vi "movimentacao_cin_inv_cubo_magico.vi"() -> ()   [LabVIEW 2017]
doc: "The myRIO Project template acquires acceleration data from the onboard accelerometer and displays the changes of acceleration values in a waveform chart."
uses:
  <vilib>/Analysis/Matrix/Datatypes/RealMatrix.ctl
  <vilib>/myRIO/Instrument Drivers/Onboard IO/PWM/typedefs/PWM Reference.ctl
  <vilib>/myRIO/Common/Instrument Driver Framework/Utilities/typedefs/myRIO Generic Hardware Reference.ctl
  <vilib>/myRIO/Common/Instrument Driver Framework/Utilities/typedefs/Hardware Version Enum.ctl
  <vilib>/myRIO/Common/Instrument Driver Framework/Utilities/typedefs/myRIO v1.0 Reference.ctl
  <vilib>/myRIO/Common/Instrument Driver Framework/Utilities/typedefs/Generic FPGA Reference.ctl
  <vilib>/myRIO/Common/Instrument Driver Framework/myRIO v1.0/PWM/typedefs/PWM Channels Enum.ctl
  <vilib>/myRIO/Instrument Drivers/Onboard IO/PWM/typedefs/PWM Configuration.ctl
  <vilib>/userdefined/High Color/nirio_resource_hc.ctl
  <vilib>/myRIO/Common/Instrument Driver Framework/myRIO v1.0/PWM/vis/myRIO v1.1 Open PWM.vi
  <vilib>/myRIO/Common/Instrument Driver Framework/Utilities/vis/Validate Channels.vi
  <vilib>/myRIO/Common/Instrument Driver Framework/myRIO v1.0/PWM/vis/myRIO v1.0 Reserve PWM.vi
  <vilib>/myRIO/Instrument Drivers/Onboard IO/PWM/vis/Set Duty Cycle and Frequency.vi
  <vilib>/myRIO/Common/Instrument Driver Framework/myRIO v1.0/PWM/vis/myRIO v1.0 Close PWM.vi
  <vilib>/myRIO/Common/Instrument Driver Framework/myRIO v1.0/PWM/vis/myRIO v1.0 Build MUX Configuration PWM.vi
  <vilib>/myRIO/Common/Instrument Driver Framework/myRIO v1.0/Resource Manager/vis/myRIO v1.0 Reserve Channel List.vi
  <vilib>/myRIO/Common/Instrument Driver Framework/myRIO v1.0/PWM/vis/myRIO v1.0 Unreserve PWM.vi
  <vilib>/myRIO/Common/Instrument Driver Framework/myRIO v1.0/Resource Manager/vis/myRIO v1.0 Create Configuration List.vi
  <vilib>/myRIO/Common/Instrument Driver Framework/myRIO v1.0/Resource Manager/vis/myRIO v1.0 Reserve Channel.vi
  <vilib>/myRIO/Common/Instrument Driver Framework/myRIO v1.0/Resource Manager/vis/myRIO v1.0 Unreserve Channel.vi
  <vilib>/myRIO/Common/Instrument Driver Framework/myRIO v1.0/Resource Manager/vis/myRIO v1.0 Unreserve Channel List.vi
  <vilib>/myRIO/Common/Instrument Driver Framework/myRIO v1.0/Resource Manager/vis/myRIO v1.0 Build Mutex Name.vi
  <vilib>/Utility/VariantDataType/GetNumericInfo.vi
  <vilib>/Utility/error.llb/Error Cluster From Error Code.vi
  <vilib>/myRIO/Common/Instrument Driver Framework/myRIO v1.0/myRIO v1.1 Open.vi
  <vilib>/myRIO/Common/Instrument Driver Framework/Utilities/vis/IO Manager.vi
  <vilib>/myRIO/Common/Instrument Driver Framework/Utilities/vis/Configuration Manager.vi
  <vilib>/myRIO/Common/Instrument Driver Framework/myRIO v1.0/Resource Manager/vis/myRIO v1.0 Configure IO.vi
  <vilib>/myRIO/Common/Instrument Driver Framework/myRIO v1.0/myRIO v1.0 Close.vi
  <vilib>/myRIO/Common/Instrument Driver Framework/myRIO v1.0/PWM/vis/myRIO v1.0 Write PWM.vi
  <vilib>/myRIO/Common/Instrument Driver Framework/myRIO v1.0/PWM/vis/myRIO v1.0 Shutdown PWM.vi
  <vilib>/myRIO/Instrument Drivers/Onboard IO/PWM/vis/myRIO PWM Open.xnode
  <vilib>/myRIO/Instrument Drivers/Onboard IO/PWM/PWM.lvlib
  <vilib>/Analysis/Matrix/NI_Matrix.lvlib
panel:
  out "Home":dbl[](array[numeric])
  out "a2 2":dbl
  out "a1 2":dbl
  out "a3 2":dbl
  out "d4 2":dbl=3.0
  in  "Array":dbl[](array[numeric])
  in  "Duty Cycle Abert 2":dbl
  in  "Actuator 3":bool
  out "punho":dbl
  in  "theta6":dbl(knob) scale=-180.0..180.0
  out "indexador 2":i32
  in  "x":i32=1
  out "antebraço":dbl
  in  "theta4":dbl(knob) scale=-180.0..180.0
  in  "matrix 2":T1=[[240.0, 240.0, 240.0], [0.0, 0.0, 0.0], [110.0, 15.0, 110.0], [-60.0, -60.0, -60.0]]
  out "subarray":dbl[](array[numeric])
  out "garra":dbl
  in  "theta5":dbl(knob) scale=-180.0..180.0
  out "output array":T1
  in  "LOCAL":T2(ring)
  in  "Duty Cycle Abert":dbl=0.04 format="%#_13g"
  out "Actuator 2":bool
  in  "Actuator":bool
  in  "Conveyor speed (mm/s)":dbl(slide)=200.0 step=1.0 scale=0.0..350.0
  out "indexador":i32
  out "Objeto detectado":bool
  in  "objeto detectado":bool
  out "Manipulando":bool
  out "Está em Home":bool
  out "Posicao_desejada":bool
  in  "Home":bool
  in  "error in (no error)":errorcluster
  in  "PARAR":bool
  out "Ângulo dos motores em graus":T3
  out "a2":dbl
  out "a1":dbl
  out "a3":dbl
  out "d4":dbl=3.0
  in  "vetor_P":dbl[](array[numeric])
  # "STATUS"
  # "OBJ.\nDET."
  # "POS.\nDES."
  # "HOM."
  # "vetor"
  # "vetor"
  # "vetor"
  # "garra"
  # "antebraço"
  # "punho"
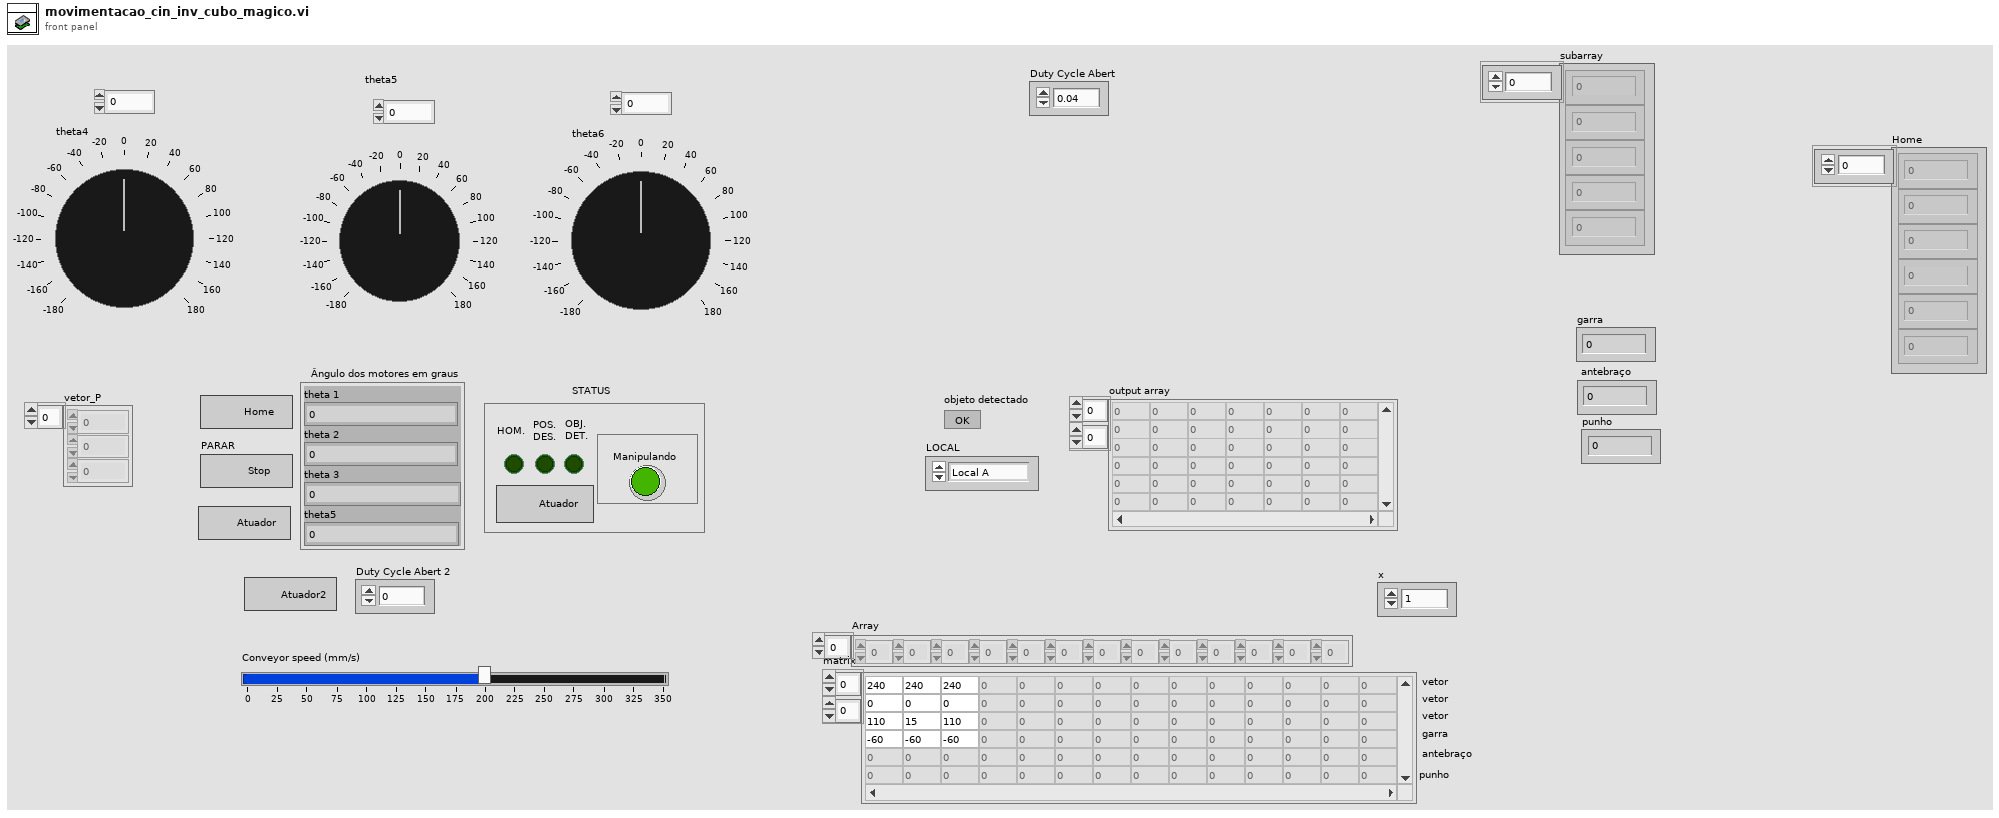
[diagram p1: front panel]
types:
  T1 = typedef "NI_Matrix.lvlib/RealMatrix.ctl" = dbl[][]
  T2 = enum16{"Local A", "Local B", "Local C", "Discard"}
  T3 = cluster{"theta 1":dbl, "theta 2":dbl, "theta 3":dbl, "theta5":dbl}
  T4 = typedef "nirio_resource_hc.ctl" = tag
  T5 = typedef "Hardware Version Enum.ctl" = enum16{"Unknown", "myRIO-1900", "myRIO-1950", "roboRIO", "NI ELVIS RIO CM"}
  T6 = typedef "PWM.lvlib/PWM Reference.ctl" = cluster{"myRIO Reference":T7, "PWM Channels Enum":T10, "PWM Configuration":T11}
  T7 = typedef "myRIO Generic Hardware Reference.ctl" = cluster{"myRIO Model":T5, "myRIO Hardware Reference":T8}
  T8 = typedef "myRIO v1.0 Reference.ctl" = cluster{"Generic FPGA Reference":T9, "Allow multiple opens":bool}
  T9 = typedef "Generic FPGA Reference.ctl" = refnum<k20>
  T10 = typedef "PWM Channels Enum.ctl" = enum16{"Not Connected", "C/PWM0", "C/PWM1", "A/PWM0", "A/PWM1", "A/PWM2", "B/PWM0", "B/PWM1", "B/PWM2", "PWM/PWM0", "PWM/PWM1", "PWM/PWM2", "PWM/PWM3", "PWM/PWM4", "PWM/PWM5", "PWM/PWM6", "PWM/PWM7", "PWM/PWM8", "PWM/PWM9"}
  T11 = typedef "PWM.lvlib/PWM Configuration.ctl" = cluster{"Frequency":dbl, "Duty Cycle":dbl}
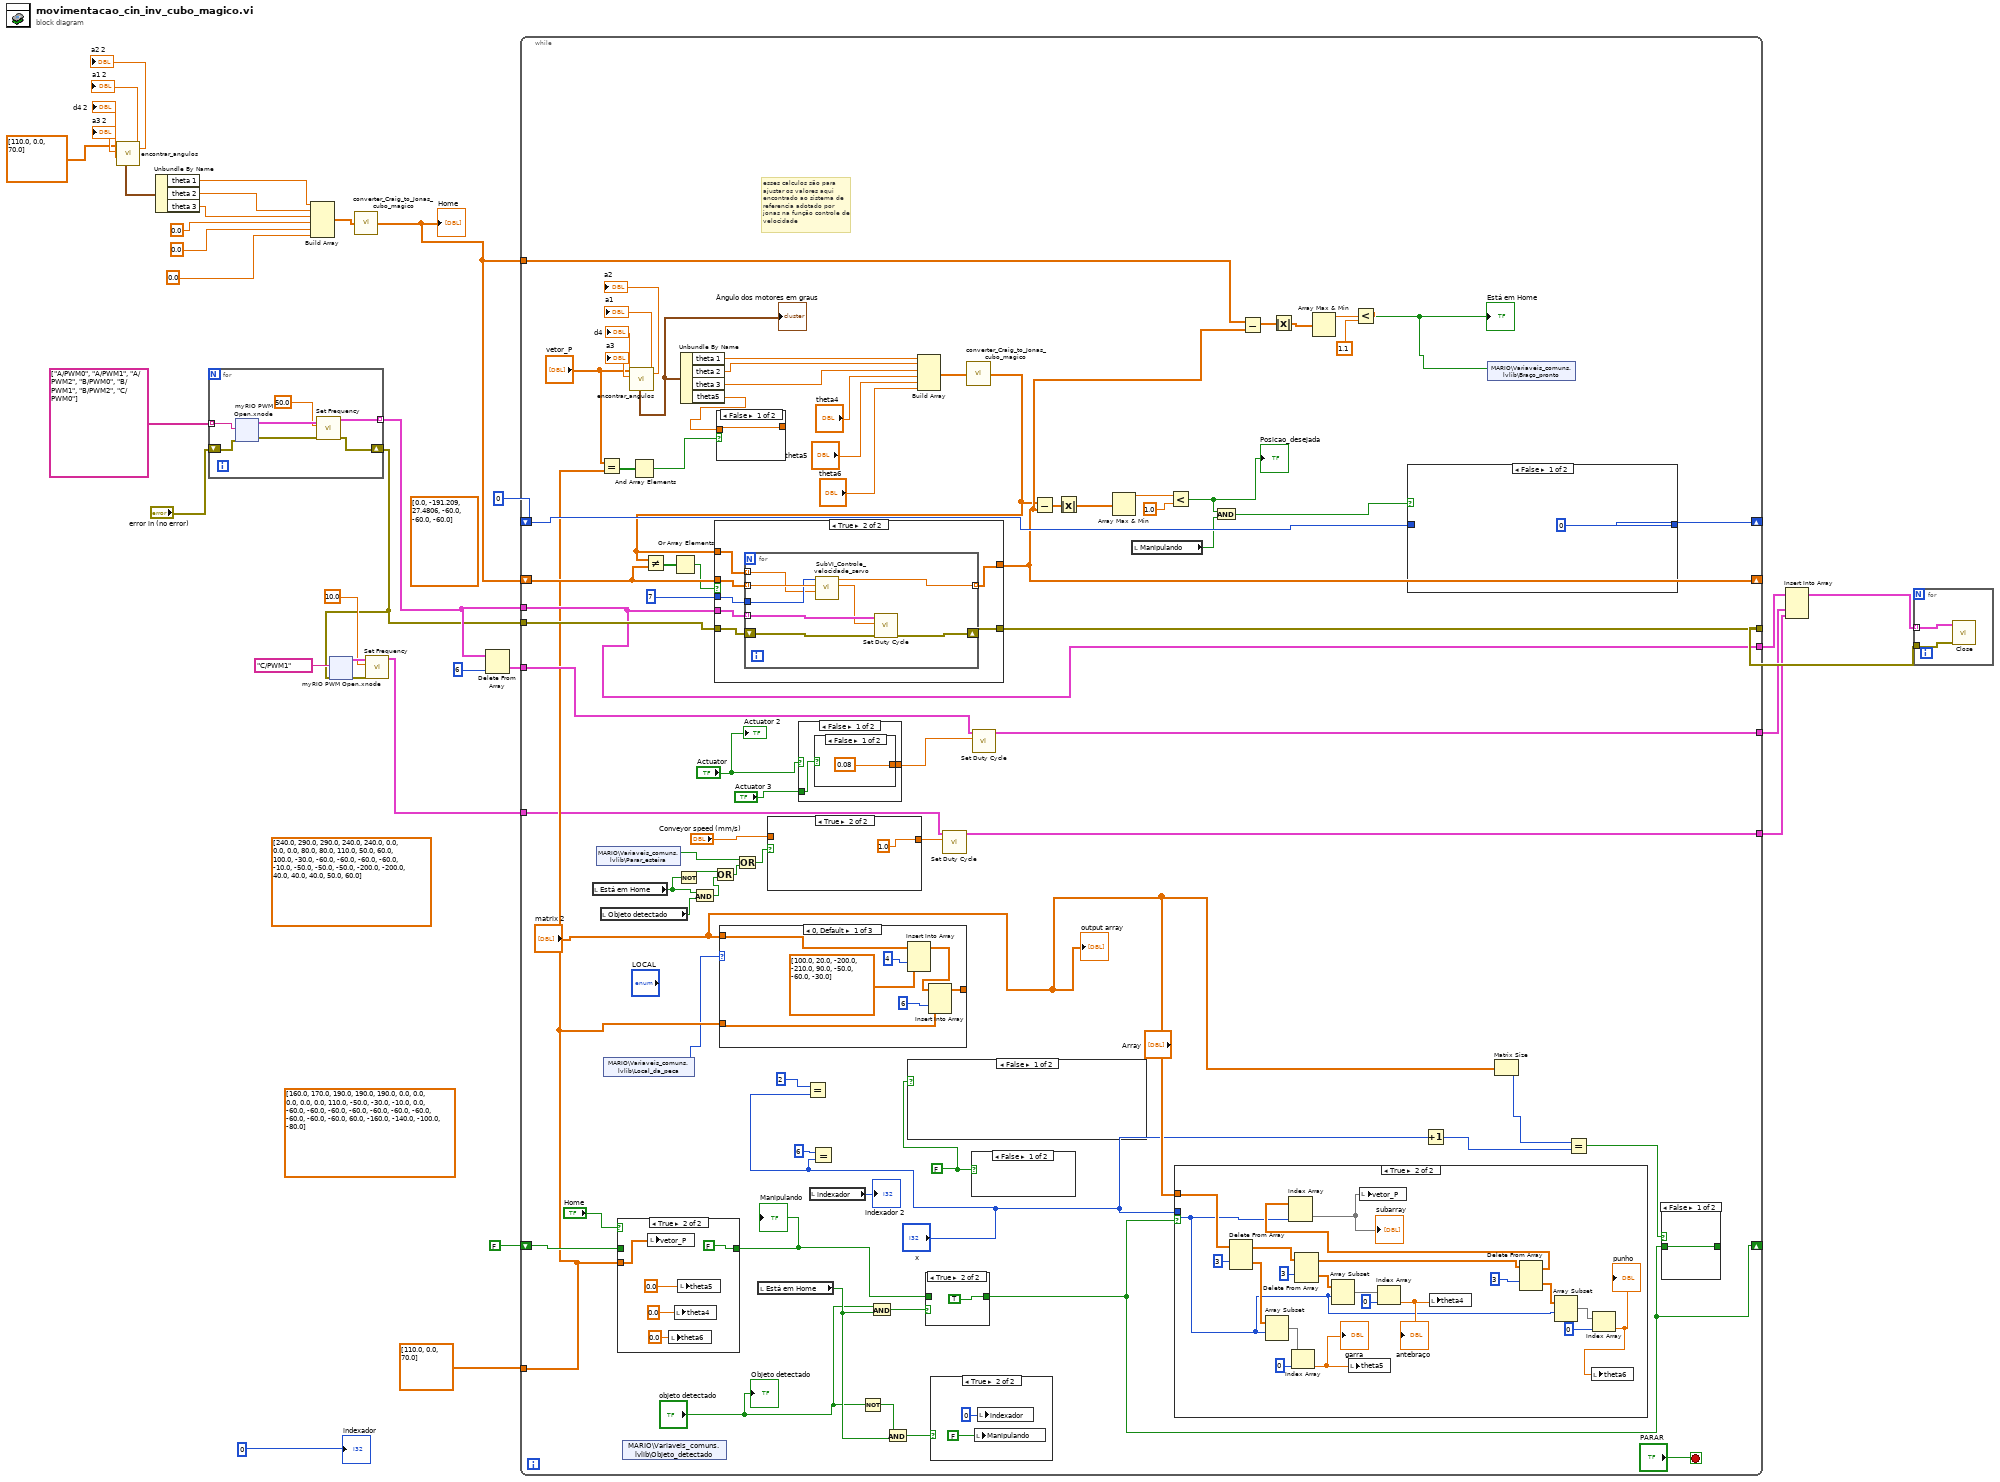
[diagram p0: block diagram]
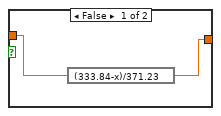
[diagram p2: hidden frame]
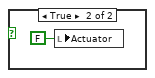
[diagram p3: hidden frame]
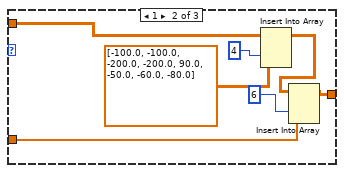
[diagram p4: hidden frame]
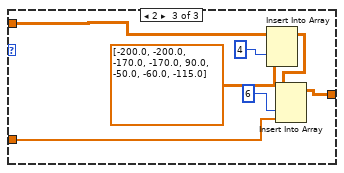
[diagram p5: hidden frame]
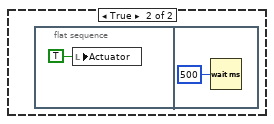
[diagram p6: hidden frame]
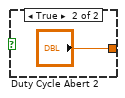
[diagram p7: hidden frame]
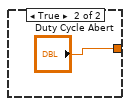
[diagram p8: hidden frame]
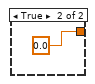
[diagram p9: hidden frame]
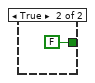
[diagram p10: hidden frame]
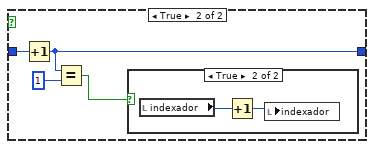
[diagram p12: hidden frame]
diagram:
  (unwired) T1 [[160.0, 170.0, 190.0, 190.0, 190.0], [0.0, 0.0, 0.0, 0.0, 0.0], [110.0, -50.0, -30.0, -10.0, 0.0], [-60.0, -60.0, -60.0, -60.0, -60.0], [-60.0, -60.0, -60.0, -60.0, -60.0], [60.0, -160.0, -140.0, -100.0, -80.0]] ("matrix 3")
  (unwired) T1 [[240.0, 290.0, 290.0, 240.0, 240.0], [0.0, 0.0, 0.0, 80.0, 80.0], [110.0, 50.0, 60.0, 100.0, -30.0], [-60.0, -60.0, -60.0, -60.0, -10.0], [-50.0, -50.0, -50.0, -200.0, -200.0], [40.0, 40.0, 40.0, 50.0, 60.0]] ("matrix 3")
  (unwired) dbl[] [0.0, -191.209, 27.4806, -60.0, -60.0, -60.0]
  n1 = call "encontrar_angulos.vi"("vetor_P"=dbl[] [110.0, 0.0, 70.0]) -> ("d4"=→"d4 2":dbl, "a3"=→"a3 2":dbl, "a1"=→"a1 2":dbl, "a2"=→"a2 2":dbl, "ângulo dos motores em graus"=w9:T3)  [unwired: 4 in, 2 out]
  n2 = Unbundle By Name(w9) -> ("theta 1"=w8:dbl, "theta 2"=w7:dbl, "theta 3"=w6:dbl)
  n3 = for {
    tunnel: tag[] ["A/PWM0", "A/PWM1", "A/PWM2", "B/PWM0", "B/PWM1", "B/PWM2", "C/PWM0"] -> [w38] mode=indexing
    tunnel: [w37] -> w28 mode=indexing
    shift-right: [w36] -> w16
    shift-left: "error in (no error)" -> [w35]
    n4 = xnode ("myRIO PWM Open.xnode")("error in (no error)"=w35, "Channel Name"=w38) -> ("error out"=w39:errorcluster, "PWM Ref Out"=w41:T6)  [unwired: 1 in]
    n5 = call <vilib>:"Set Frequency.vi"("error in (no error)"=w39, "Frequency [Hz]"=50.0, "PWM Ref In"=w41) -> ("error out"=w36:errorcluster, "PWM Ref Out"=w37:T6)  [unwired: 6 in]
  }
  n6 = Build Array(w8, w7, w6, 0.0, 0.0, 0.0) -> (w2:dbl[])
  n7 = xnode "myRIO PWM Open.xnode"("error in (no error)"=w16, "Channel Name"=tag "C/PWM1") -> ("error out"=w20:errorcluster, "PWM Ref Out"=w21:T6)  [unwired: 1 in]
  n8 = call "converter_Craig_to_Jonas_cubo_magico.vi"("Craig"=w2) -> ("Jonas"=w1:dbl[])
  "Home" <- w1
  n9 = call <vilib>:"Set Frequency.vi"("error in (no error)"=w20, "Frequency [Hz]"=10.0, "PWM Ref In"=w21) -> ("PWM Ref Out"=w17:T6)  [unwired: 6 in, 1 out]
  n10 = Delete From Array(array=w28, index=6) -> (deleted portion=w26:T6)  [unwired: 1 in, 1 out]
  n11 = while {
    tunnel: [w133] -> w34
    shift-right: [w109] -> _
    shift-left: w1 -> [w132]
    tunnel: w16 -> [w130]
    tunnel: w28 -> [w129]
    tunnel: [w129] -> w25
    tunnel: dbl[] [110.0, 0.0, 70.0] -> [w90]
    shift-right: [w68] -> _
    shift-left: FALSE -> [w104]
    shift-right: [w115] -> _
    shift-left: u32 0 ("ms to wait (braço)") -> [w114]
    tunnel: w26 -> [w94]
    tunnel: [w93] -> w24
    tunnel: w17 -> [w88]
    tunnel: [w84] -> w15
    tunnel: w1 -> [w58]
    stop <- "PARAR" stop-if-true
    w69 = FALSE
    # "esses calculos são para ajustar os valores aqui encontrado ao sistema de referencia adotado por jonas na função controle de velocidade"
    n12 = local read "Está em Home"() -> (w78:bool)
    n13 = shared-variable "MARIO\\Variaveis_comuns.lvlib\\Parar_esteira"() -> (w83:bool)  [unwired: 1 in, 1 out]
    n14 = Equal?(x="vetor_P", y=w90) -> (x = y?=w97:bool[])
    n15 = local read "Objeto detectado"() -> (w81:bool)
    n16 = shared-variable "MARIO\\Variaveis_comuns.lvlib\\Local_da_peca"() -> (w76:i8)  [unwired: 1 in, 1 out]
    n17 = case shown="True" "Home" {
      tunnel: w90 -> [_ w208]
      tunnel: w104 -> [w203 _]
      tunnel: [w203 FALSE ("Manipulando")] -> w99
      frame False {
      }
      frame True {
        n18 = local write "vetor_P"(w208) -> ()
        n19 = local write "theta6"(0.0 ("punho")) -> ()
        n20 = local write "theta4"(0.0 ("antebraço")) -> ()
        n21 = local write "theta5"(0.0 ("angulo_garra")) -> ()
      }
    }
    "Manipulando" <- w99
    n22 = shared-variable "MARIO\\Variaveis_comuns.lvlib\\Objeto_detectado"() -> ()  [unwired: 1 in, 2 out]
    n23 = call "encontrar_angulos.vi"("vetor_P"="vetor_P") -> ("d4"=→"d4":dbl, "a3"=→"a3":dbl, "a1"=→"a1":dbl, "a2"=→"a2":dbl, "ângulo dos motores em graus"=w128:T3)  [unwired: 4 in, 2 out]
    "Ângulo dos motores em graus" <- w128
    n24 = And Array Elements(Boolean array=w97) -> (logical AND=w96:bool)
    n25 = Not(x=w78) -> (.not. x?=w79:bool)
    n26 = Unbundle By Name(w128) -> ("theta 1"=w66:dbl, "theta 2"=w65:dbl, "theta 3"=w64:dbl, "theta5"=w75:dbl)
    n27 = And(x=w78, y=w81) -> (x .and. y?=w80:bool)
    n28 = Or(x=w79, y=w80) -> (x .or. y?=w77:bool)
    n29 = case shown="False" w96 {
      tunnel: [w167 0.0 ("theta5")] -> _
      tunnel: w75 -> [w167 _]
      frame False {
      }
      frame True {
      }
    }
    n30 = case shown="0, Default" w76 {
      tunnel: "matrix 2" -> [w139 w148 w156]
      tunnel: w90 -> [w141 w147 w155]
      tunnel: [w140 w146 w154] -> _
      frame 0, Default {
        n31 = Insert Into Array(array=w139, index (col)=4 ("disabled index (col)"), new element=T1 [[100.0, 20.0], [-200.0, -210.0], [90.0, -50.0], [-60.0, -30.0]] ("matrix")) -> (w143:T1)  [unwired: 1 in]
        n32 = Insert Into Array(array=w143, index (col)=6 ("disabled index (col)"), new element=w141) -> (w140:T1)  [unwired: 1 in]
      }
      frame 1 {
        n33 = Insert Into Array(array=w148, index (col)=4 ("disabled index (col)"), new element=T1 [[-100.0, -100.0], [-200.0, -200.0], [90.0, -50.0], [-60.0, -80.0]] ("matrix")) -> (w150:T1)  [unwired: 1 in]
        n34 = Insert Into Array(array=w150, index (col)=6 ("disabled index (col)"), new element=w147) -> (w146:T1)  [unwired: 1 in]
      }
      frame 2 {
        n35 = Insert Into Array(array=w156, index (col)=4 ("disabled index (col)"), new element=T1 [[-200.0, -200.0], [-170.0, -170.0], [90.0, -50.0], [-60.0, -115.0]] ("matrix")) -> (w153:T1)  [unwired: 1 in]
        n36 = Insert Into Array(array=w153, index (col)=6 ("disabled index (col)"), new element=w155) -> (w154:T1)  [unwired: 1 in]
      }
    }
    n37 = Or(x=w83, y=w77) -> (x .or. y?=w85:bool)
    n38 = local read "Está em Home"() -> (w103:bool)
    n39 = case shown="True" w85 {
      tunnel: [w136 1.0 ("Duty Cycle")] -> w87
      tunnel: "Conveyor speed (mm/s)" -> [w135 _]
      frame False {
        n40 = expression code="(333.84-x)/371.23"(w135) -> (w136:dbl)
      }
      frame True {
      }
    }
    n41 = case shown="False" "Actuator" {
      tunnel: [w163 "Duty Cycle Abert"] -> w92
      tunnel: "Actuator 3" -> [w162 _]
      frame False {
        n42 = case shown="False" w162 {
          tunnel: [0.08 ("Duty Cycle Abert") "Duty Cycle Abert 2"] -> w163
          frame False {
          }
          frame True {
          }
        }
      }
      frame True {
      }
    }
    n43 = Equal?(x=2, y="x") -> ()  [unwired: 1 out]
    n44 = local read "indexador"() -> (→"indexador 2":i32)
    n45 = Equal?(x=6, y="x") -> ()  [unwired: 1 out]
    n46 = Not(x="objeto detectado") -> (.not. x?=w102:bool)
    n47 = And(x="objeto detectado", y=w103) -> (x .and. y?=w117:bool)
    n48 = And(x=w102, y=w103) -> (x .and. y?=w111:bool)
    n49 = case shown="False" w69 {
      frame False {
      }
      frame True {
        n50 = flat-sequence {
          frame #0 {
            n51 = local write "Actuator"(TRUE ("Actuator")) -> ()
          }
          frame #1 {
            n52 = Wait (ms)(milliseconds to wait=u32 500) -> ()  [unwired: 1 out]
          }
        }
      }
    }
    n53 = Build Array(w66, w65, w64, "theta4", "theta5", "theta6") -> (w60:dbl[])
    n54 = case shown="True" w117 {
      tunnel: [w201 TRUE] -> w68
      tunnel: w99 -> [w201 _]
      frame False {
      }
      frame True {
      }
    }
    n55 = case shown="True" w111 {
      frame False {
      }
      frame True {
        n56 = local write "Manipulando"(FALSE ("Manipulando")) -> ()
        n57 = local write "indexador"(0 ("indexador")) -> ()
      }
    }
    n58 = call <vilib>:"Set Duty Cycle.vi"("Duty Cycle"=w87, "PWM Ref In"=w88) -> ("PWM Ref Out"=w84:T6)  [unwired: 7 in, 1 out]
    n59 = call "converter_Craig_to_Jonas_cubo_magico.vi"("Craig"=w60) -> ("Jonas"=w59:dbl[])
    n60 = Not Equal?(x=w59, y=w132) -> (x != y?=w123:bool[])
    n61 = Or Array Elements(Boolean array=w123) -> (logical OR=w122:bool)
    n62 = case shown="True" w122 {
      tunnel: [w209 w217] -> w133
      tunnel: w130 -> [w209 w216]
      tunnel: w129 -> [_ w215]
      tunnel: w132 -> [w210 w214]
      tunnel: [w210 w212] -> w109
      tunnel: u32 7 ("ms to wait (braço)") -> [_ w213]
      tunnel: w59 -> [_ w211]
      frame False {
      }
      frame True {
        n63 = for {
          tunnel: w215 -> [w223] mode=indexing
          tunnel: w214 -> [w222] mode=indexing
          tunnel: w213 -> [w220]
          tunnel: [w219] -> w212 mode=indexing
          tunnel: w211 -> [w218] mode=indexing
          shift-right: [w225] -> w217
          shift-left: w216 -> [w224]
          n64 = call "SubVI_Controle_velocidade_servo.vi"("Posição Desejada"=w218, "Posição"=w222, "milliseconds to wait"=w220) -> ("Duty Cycle"=w221:dbl, "Posição"=w219:dbl)  [unwired: 7 in]
          n65 = call <vilib>:"Set Duty Cycle.vi"("error in (no error)"=w224, "Duty Cycle"=w221, "PWM Ref In"=w223) -> ("error out"=w225:errorcluster)  [unwired: 6 in, 1 out]
        }
      }
    }
    n66 = case shown="False" w69 {
      frame False {
      }
      frame True {
        n67 = local write "Actuator"(FALSE ("Actuator")) -> ()
      }
    }
    n68 = call <vilib>:"Set Duty Cycle.vi"("Duty Cycle"=w92, "PWM Ref In"=w94) -> ("PWM Ref Out"=w93:T6)  [unwired: 7 in, 1 out]
    n69 = Subtract(x=w59, y=w109) -> (x-y=w121:dbl[])
    n70 = Absolute Value(x=w121) -> (abs(x)=w120:dbl[])
    n71 = Array Max & Min(array=w120) -> (max value=w119:dbl)  [unwired: 3 out]
    n72 = local read "Manipulando"() -> (w113:bool)
    n73 = Less?(x=w119, y=1.0) -> (x < y?=w110:bool)
    "Posicao_desejada" <- w110
    n74 = case shown="True" w68 {
      tunnel: "matrix 2" -> [_ w190]
      tunnel: "x" -> [_ w174]
      frame False {
      }
      frame True {
        n75 = Delete From Array(array=w190, index (row)=3) -> (deleted portion=w188:dbl[], array with subset deleted=w183:T1)  [unwired: 2 in]
        n76 = Array Subset(array=w188, index=w174) -> (w187:dbl[])  [unwired: 1 in]
        n77 = Index Array(array=w187, index=0) -> (element=w185:dbl)
        "garra" <- w185
        n78 = Delete From Array(array=w183, index (row)=3) -> (deleted portion=w182:dbl[], array with subset deleted=w177:T1)  [unwired: 2 in]
        n79 = Array Subset(array=w182, index=w174) -> (w181:dbl[])  [unwired: 1 in]
        n80 = local write "theta5"(w185) -> ()
        n81 = Index Array(array=w181, index=0) -> (element=w179:dbl)
        "antebraço" <- w179
        n82 = local write "theta4"(w179) -> ()
        n83 = Delete From Array(array=w177, index (row)=3 ("index (col)")) -> (deleted portion=w175:dbl[], array with subset deleted=w176:T1)  [unwired: 2 in]
        n84 = Index Array(array=w176, index (col)=w174) -> (element=w191:dbl[])  [unwired: 1 in]
        "subarray" <- w191
        n85 = local write "vetor_P"(w191) -> ()
        n86 = Array Subset(array=w175, index=w174) -> (w173:dbl[])  [unwired: 1 in]
        n87 = Index Array(array=w173, index=0) -> (element=w171:dbl)
        "punho" <- w171
        n88 = local write "theta6"(w171) -> ()
      }
    }
    n89 = And(x=w110, y=w113) -> (x .and. y?=w112:bool)
    n90 = Subtract(x=w58, y=w109) -> (x-y=w108:dbl[])
    n91 = Absolute Value(x=w108) -> (abs(x)=w107:dbl[])
    n92 = Array Max & Min(array=w107) -> (max value=w106:dbl)  [unwired: 3 out]
    n93 = Less?(x=w106, y=1.1) -> (x < y?=w82:bool)
    "Está em Home" <- w82
    n94 = case shown="False" w112 {
      tunnel: w114 -> [_ w196]
      tunnel: [u32 0 ("ms to wait (braço)") w195] -> w115
      frame False {
      }
      frame True {
        n95 = Increment(x=w196) -> (x+1=w195:u32)
        n96 = Equal?(x=w195, y=u32 1) -> (x = y?=w193:bool)
        n97 = case shown="True" w193 {
          frame False {
          }
          frame True {
            n98 = local read "indexador"() -> (w198:i32)
            n99 = Increment(x=w198) -> (x+1=w197:i32)
            n100 = local write "indexador"(w197) -> ()
          }
        }
      }
    }
    n101 = Increment(x="x") -> (x+1=w100:i32)
    n102 = shared-variable "MARIO\\Variaveis_comuns.lvlib\\Braço_pronto"(w82) -> ()  [unwired: 1 in, 1 out]
    n103 = Matrix Size(0:"matrix 2") -> (2:w101:i32)  [unwired: 1 out]
    n104 = Equal?(x=w101, y=w100) -> (x = y?=w98:bool)
    n105 = case shown="False" w98 {
      tunnel: [w169 FALSE ("Manipulando")] -> _
      tunnel: w68 -> [w169 _]
      frame False {
      }
      frame True {
      }
    }
    "Objeto detectado" <- "objeto detectado"
    "Actuator 2" <- "Actuator"
    "output array" <- "matrix 2"
  }
  n106 = Insert Into Array(array=w25, new element #1=w24, new element #2=w15) -> (w23:T6[])  [unwired: 1 in]
  n107 = for {
    tunnel: w34 -> [w227]
    tunnel: w23 -> [w226] mode=indexing
    n108 = call <vilib>:"Close.vi"("error in (no error)"=w227, "PWM Ref In"=w226) -> ()  [unwired: 9 in, 1 out]
  }
  "indexador" <- 0
